vi "Read Buffer Statistic.vi"(0 "VISA resource name":refnum<visa-resource-name>, 7 "Statistic (0: Max)":u16(ring) items=["Max", "Min", "Mean", "Standard Deviation", "Peak to Peak"], 11 "error in (no error)":errorcluster) -> (3 "Buffer Statistic":dbl, 4 "VISA resource name out":refnum<visa-resource-name>, 15 "error out":errorcluster)   [LabVIEW 2020, in "Keithley 648X Series.lvlib"]
doc: "Reads one of the statistical properties of the data buffer."
uses:
  <instrlib>/Keithley 648X Series/Keithley 648X Series.lvlib
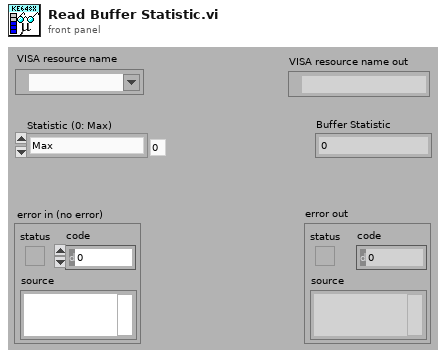
[diagram p1: front panel]
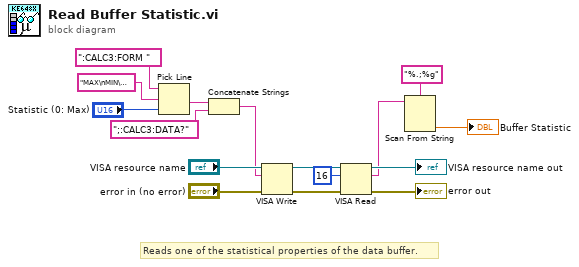
[diagram p0: block diagram]
diagram:
  # "Reads one of the statistical properties of the data buffer."
  n1 = Pick Line(string ("")=":CALC3:FORM ", multi-line string="MAX\nMIN\nMEAN\nSDEV\nPKPK", line index="Statistic (0: Max)") -> (output string=w5:string)
  n2 = Concatenate Strings(w5, ";:CALC3:DATA?" ("string")) -> (w3:string)
  n3 = VISA Write(VISA resource name="VISA resource name", write buffer=w3, error in (no error)="error in (no error)") -> (VISA resource name out=w11:refnum<visa-resource-name>, error out=w14:errorcluster)  [unwired: 1 out]
  n4 = VISA Read(VISA resource name=w11, byte count=u32 16, error in (no error)=w14) -> (VISA resource name out=→"VISA resource name out":refnum<visa-resource-name>, read buffer=w7:string, error out=→"error out":errorcluster)  [unwired: 1 out]
  n5 = Scan From String(format string="%.;%g", input string=w7) -> (output 1=→"Buffer Statistic":dbl)  [unwired: 3 in, 3 out]
